vi "Check Selected Palette in Menu.vi"(8 "Error In":errorcluster, 9 "Palette List":string[](array[string])=["Not a palette"], 10 "Checked Palette":string, 11 "Menu in":refnum<k9>) -> (0 "Error Out":errorcluster, 1 "Stored Palette List":string[](array[string]), 3 "menu reference out":refnum<k9>)   [LabVIEW 2021, in "Palette.lvlib"]
uses:
  Palette.lvlib
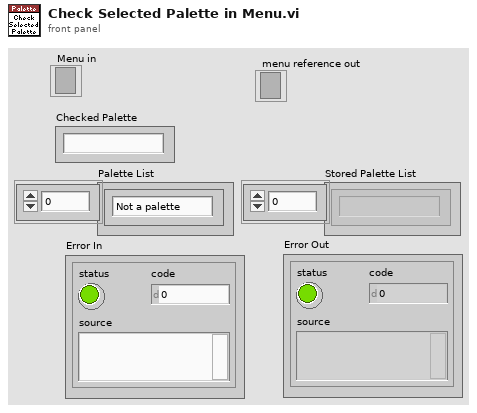
[diagram p1: front panel]
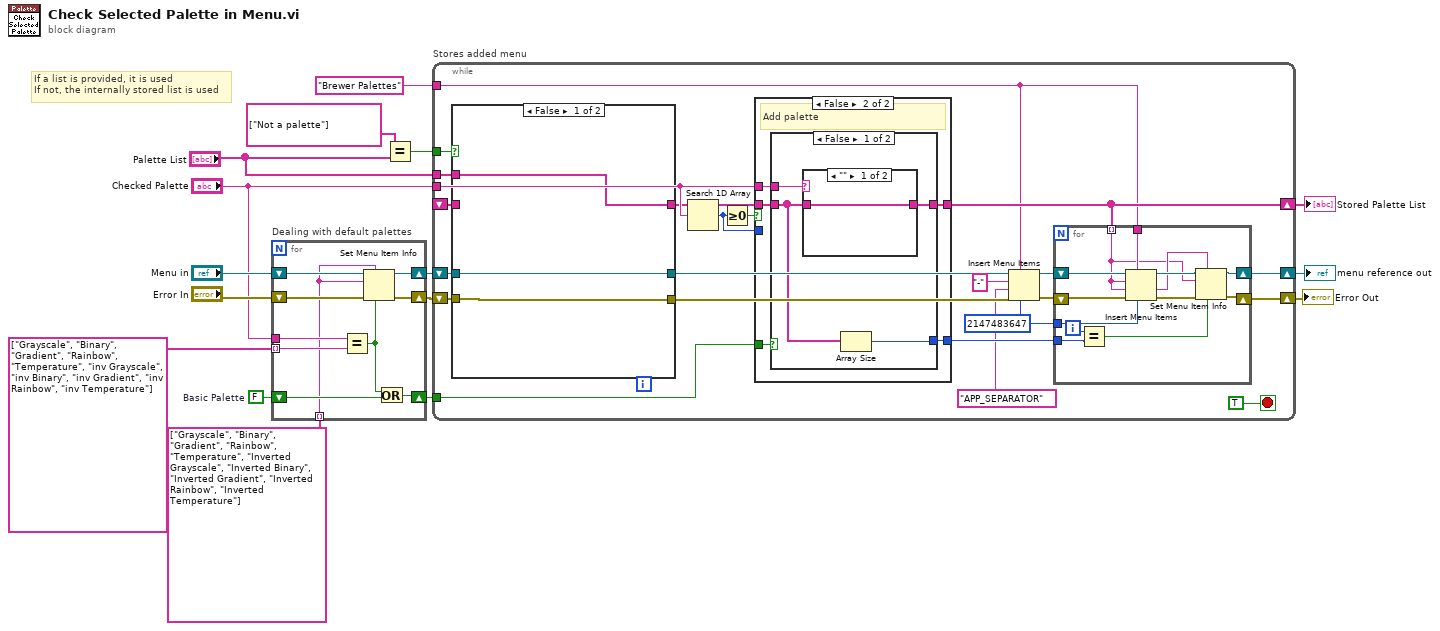
[diagram p0: block diagram]
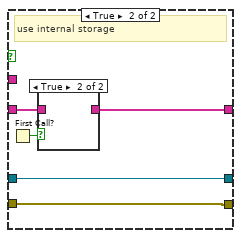
[diagram p2: hidden frame]
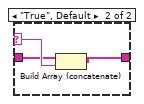
[diagram p5: hidden frame]
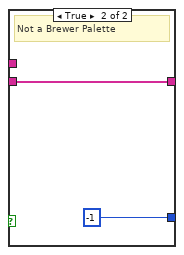
[diagram p6: hidden frame]
diagram:
  w9 = FALSE  # Basic Palette
  # "If a list is provided, it is used\nIf not, the internally stored list is used"
  n1 = for "Dealing with default palettes" {
    shift-right: [w25] -> w13
    shift-left: "Menu in" -> [w26]
    shift-right: [w23] -> w12
    shift-left: "Error In" -> [w24]
    tunnel: string[] ["Grayscale", "Binary", "Gradient", "Rainbow", "Temperature", "inv Grayscale", "inv Binary", "inv Gradient", "inv Rainbow", "inv Temperature"] ("Checked Palette") -> [w21] mode=indexing
    tunnel: "Checked Palette" -> [w22]
    shift-right: [w18] -> w8
    shift-left: w9 -> [w19]
    tunnel: string[] ["Grayscale", "Binary", "Gradient", "Rainbow", "Temperature", "Inverted Grayscale", "Inverted Binary", "Inverted Gradient", "Inverted Rainbow", "Inverted Temperature"] ("Checked Palette") -> [w17] mode=indexing
    n2 = Equal?(x=w22, y=w21) -> (x = y?=w20:bool)
    n3 = Set Menu Item Info(6:w20, 7:w17, 8:w24, 10:w17, 11:w26) -> (0:w23:errorcluster, 3:w25:refnum<k9>)  [unwired: 2 in]
    n4 = Or(x=w20, y=w19) -> (x .or. y?=w18:bool)
  }
  n5 = Equal?(x=string[] ["Not a palette"] ("Palette List"), y="Palette List") -> (x = y?=w3:bool)
  n6 = while "Stores added menu" {
    tunnel: "Checked Palette" -> [w48]
    tunnel: w8 -> [w44]
    shift-right: [w49] -> w11
    shift-left: w12 -> [w34]
    tunnel: "Brewer Palettes" ("item tag") -> [w30]
    shift-right: [w43] -> w6
    shift-left: _ -> [w40]
    shift-right: [w47] -> w2
    shift-left: w13 -> [w36]
    tunnel: w3 -> [w38]
    tunnel: "Palette List" -> [w37]
    stop <- TRUE stop-if-true
    w27 = 2147483647
    n7 = case shown="False" w38 {
      tunnel: w40 -> [_ w56]
      tunnel: [w52 w55] -> w39
      tunnel: w37 -> [w52 _]
      tunnel: w36 -> [w51 w54]
      tunnel: [w51 w54] -> w35
      tunnel: w34 -> [w50 w53]
      tunnel: [w50 w53] -> w32
      frame False {
      }
      frame True {
        # "use internal storage"
        n8 = First Call?() -> (First Call?: T/F=w57:bool)
        n9 = case shown="True" w57 {
          tunnel: w56 -> [w58 _]
          tunnel: [w58 _] -> w55
          frame False {
          }
          frame True {
          }
        }
      }
    }
    n10 = Search 1D Array(1D array=w39, element=w48) -> (index of element=w42:i32)  [unwired: 1 in]
    n11 = Greater Or Equal To 0?(x=w42) -> (x >= 0?=w45:bool)
    n12 = case shown="False" w45 {
      tunnel: w39 -> [w73 w76]
      tunnel: w48 -> [_ w78]
      tunnel: [w73 w77] -> w43
      tunnel: [w72 w75] -> w46
      tunnel: w44 -> [_ w74]
      tunnel: w42 -> [w72 _]
      frame True {
        # "Palette exists already"
      }
      frame False {
        # "Add palette"
        n13 = case shown="False" w74 {
          tunnel: w78 -> [w82 _]
          tunnel: [w81 w88] -> w77
          tunnel: w76 -> [w80 w88]
          tunnel: [w79 -1] -> w75
          frame False {
            n14 = case shown="\"\"" w82 {
              selector: w82 -> [_ w86]
              tunnel: [w83 w85] -> w81
              tunnel: w80 -> [w83 w84]
              frame "" {
              }
              frame "True", Default {
                n15 = Build Array (concatenate)(w84, w86) -> (w85:string[])
              }
            }
            n16 = Array Size(array=w80) -> (size(s)=w79:i32)
          }
          frame True {
            # "Not a Brewer Palette"
          }
        }
      }
    }
    n17 = Insert Menu Items(4:w27, 5:w30, 6:w32, 7:"APP_SEPARATOR" ("Checked Palette"), 8:"-" ("Checked Palette"), 9:w35) -> (0:w31:errorcluster, 3:w33:refnum<k9>)  [unwired: 1 out]
    n18 = for {
      tunnel: w30 -> [w70]
      tunnel: w43 -> [w65] mode=indexing
      shift-right: [w64] -> w47
      shift-left: w33 -> [w66]
      tunnel: w46 -> [w63]
      shift-right: [w71] -> w49
      shift-left: w31 -> [w60]
      tunnel: w27 -> [w59]
      i -> [w62]
      n19 = Equal?(x=w62, y=w63) -> (x = y?=w61:bool)
      n20 = Insert Menu Items(4:w59, 5:w70, 6:w60, 7:w65, 8:w65, 9:w66) -> (0:w69:errorcluster, 1:w67:string, 3:w68:refnum<k9>)
      n21 = Set Menu Item Info(6:w61, 7:w67, 8:w69, 10:w65, 11:w68) -> (0:w71:errorcluster, 3:w64:refnum<k9>)  [unwired: 2 in]
    }
  }
  "Error Out" <- w11
  "Stored Palette List" <- w6
  "menu reference out" <- w2
